vi "Teste Substrato Flexível 0.1_2022.vi"() -> ()   [LabVIEW 2016]
panel:
  out "F (Hz)":dbl format="%#_3g"
  out "Ciclos por segundo":dbl format="%#_3g"
  out "Tempo (s)":u32
  out "init":u32
  out "In LOOP":bool
  out "F2":bool
  out "F1":bool
  out "Close":bool
  out "Open":bool
  in  "Flush":bool
  in  "Loop Stop":i32=50 min=1
  in  "Loop Stop":bool
  in  "stop":bool
  in  "Loop Infinito":bool
  out "Vel Cte":i32
  in  "Vel Loop":i32(slide)=20 min=10 max=100 step=5 scale=10.0..100.0
  in  "Jog":i32=10
  in  "Jog_s":string="10"
  in  "Desl_s":string="50"
  out "Contador":dbl format="%.2f"
  in  "Power Off":bool
  in  "Down":bool
  in  "Up":bool
  out "read buffer":string
  out "Direcção":bool
  out "error":errorcluster
  in  "Arduino":refnum<visa-resource-name>="COM3"
  # "Controle Mecanismo Teste de Substrato Flexível"
  # "LOEM"
  # "Velocidade de Deslocamento"
  # "Contador de Ciclos"
  # "Parar em ciclo"
  # "CONTROLE MANUAL"
  # "Pg Up"
  # "Pg Down"
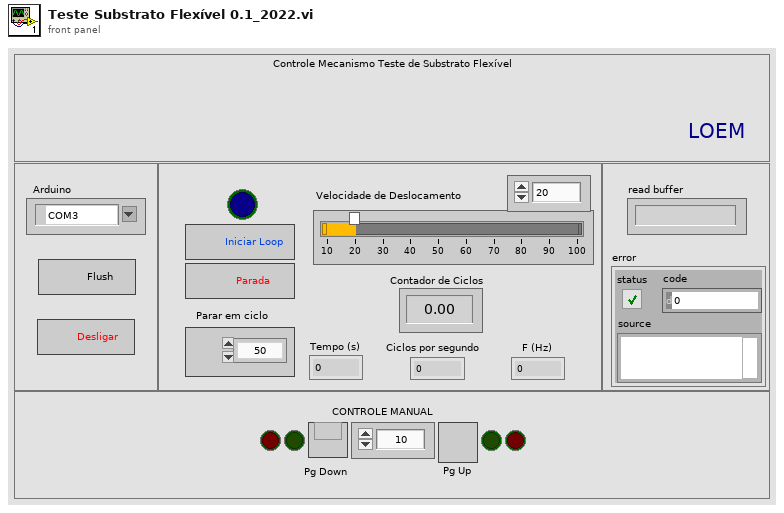
[diagram p1: front panel]
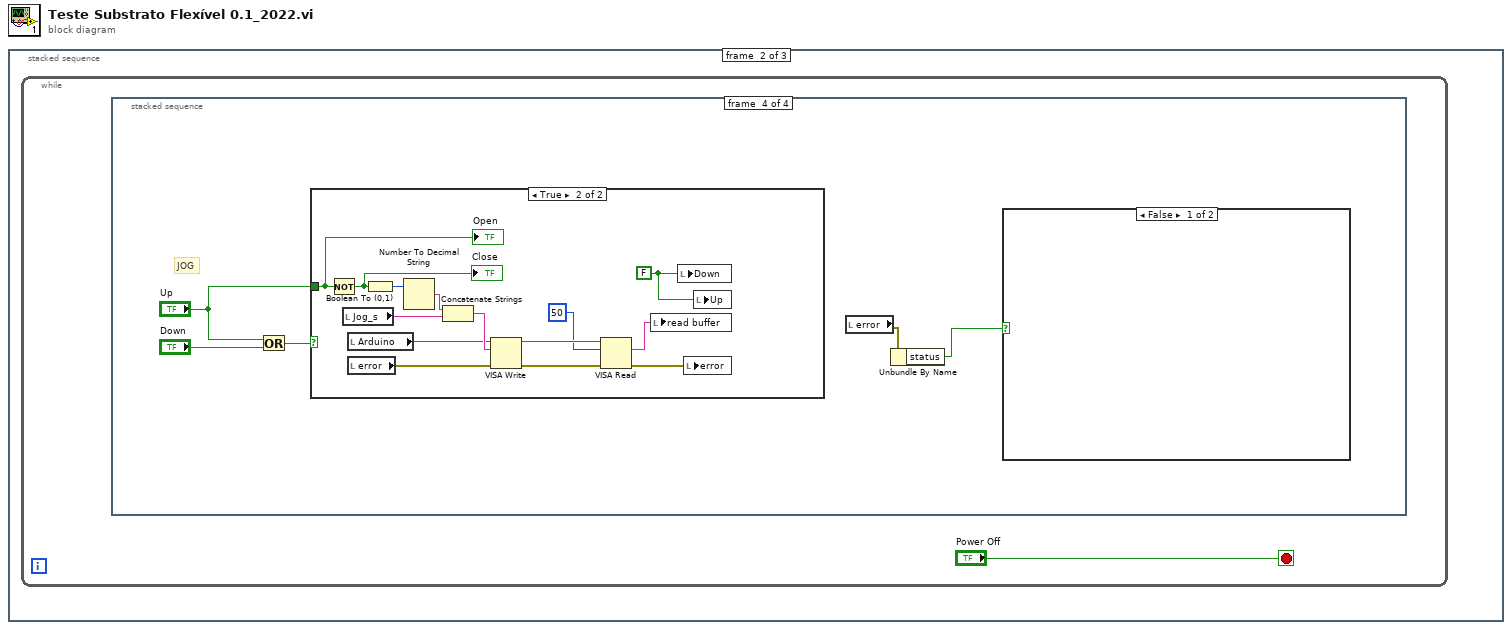
[diagram p0: block diagram]
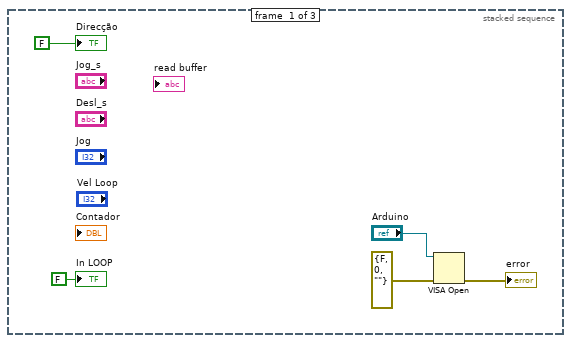
[diagram p2: hidden frame]
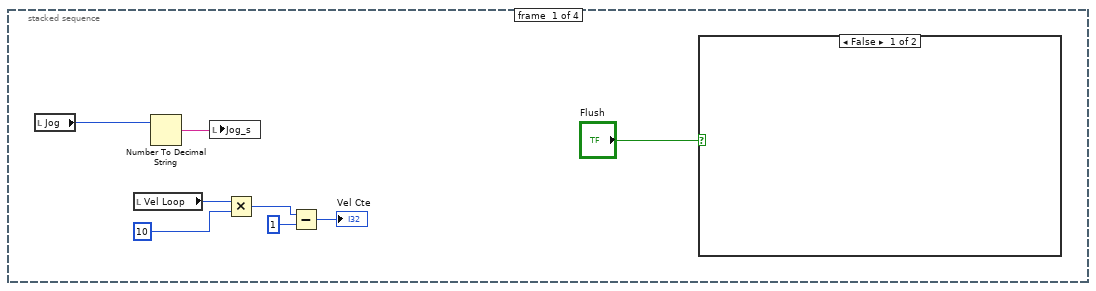
[diagram p3: hidden frame]
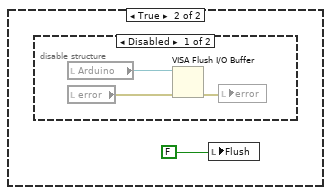
[diagram p4: hidden frame]
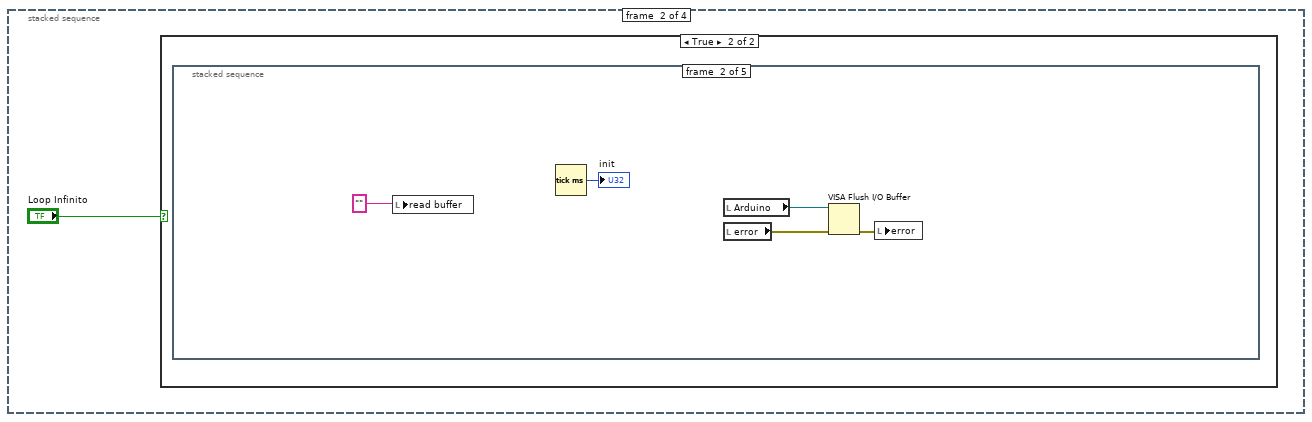
[diagram p6: hidden frame]
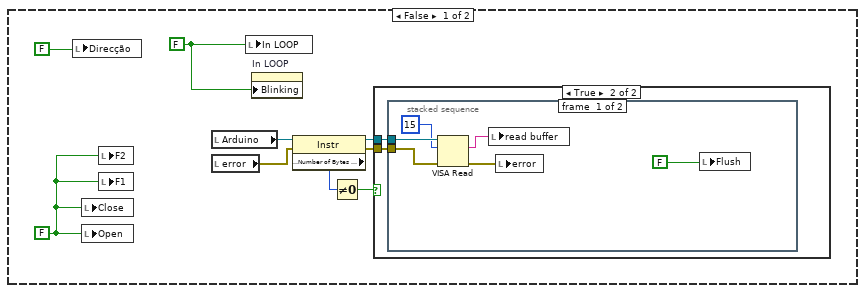
[diagram p7: hidden frame]
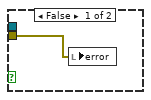
[diagram p8: hidden frame]
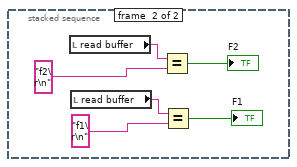
[diagram p9: hidden frame]
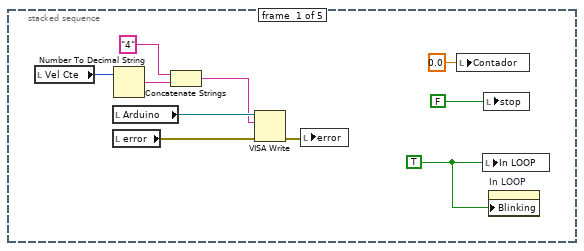
[diagram p10: hidden frame]
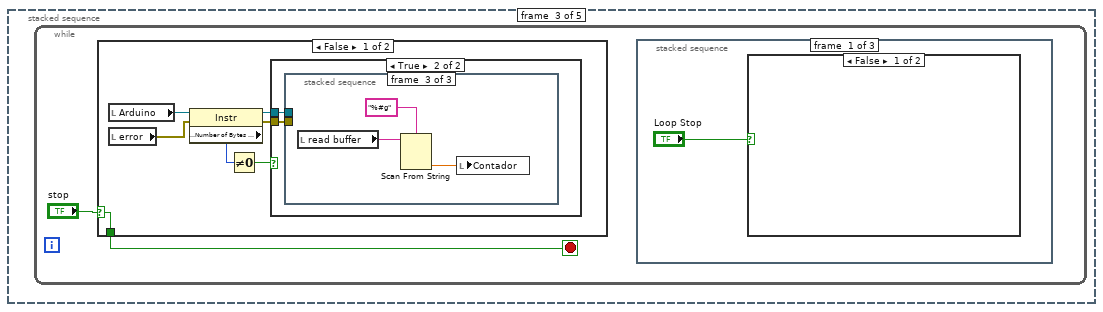
[diagram p11: hidden frame]
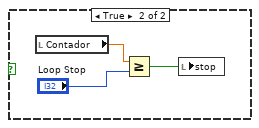
[diagram p12: hidden frame]
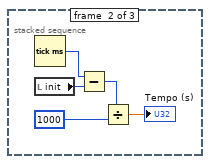
[diagram p13: hidden frame]
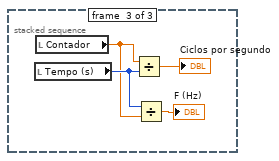
[diagram p14: hidden frame]
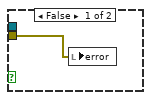
[diagram p15: hidden frame]
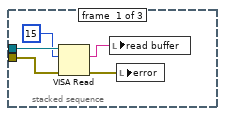
[diagram p16: hidden frame]
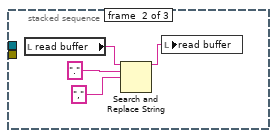
[diagram p17: hidden frame]
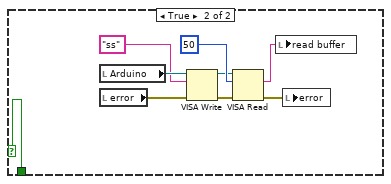
[diagram p18: hidden frame]
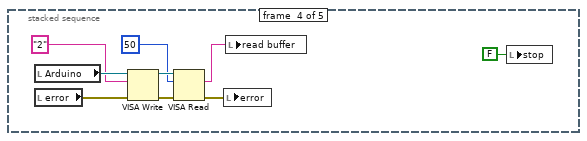
[diagram p19: hidden frame]
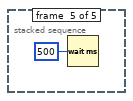
[diagram p20: hidden frame]
diagram:
  n1 = stacked-sequence {
    frame #0 {
      n2 = VISA Open(error in (no error)=errorcluster {"status"=FALSE, "code"=0, "source"=""}, VISA resource name="Arduino") -> (error out=→"error":errorcluster)  [unwired: 3 in, 1 out]
      "Direcção" <- FALSE ("Direcção")
      "In LOOP" <- FALSE ("In LOOP")
    }
    frame #1 {
      n3 = while {
        stop <- "Power Off" stop-if-true
        n4 = stacked-sequence {
          frame #0 {
            n5 = local read "Jog"() -> (w14:i32)
            n6 = local read "Vel Loop"() -> (w11:i32)
            n7 = Number To Decimal String(number=w14) -> (decimal integer string=w13:string)  [unwired: 1 in]
            n8 = local write "Jog_s"(w13) -> ()
            n9 = Multiply(x=w11, y=10) -> (x*y=w12:i32)
            n10 = Subtract(x=w12, y=1) -> (x-y=→"Vel Cte":i32)
            n11 = case shown="False" "Flush" {
              frame False {
              }
              frame True {
                n12 = disable-structure shown="Disabled" {
                  frame Disabled {
                    n13 = local read "Arduino"() -> (w16:refnum<visa-resource-name>)
                    n14 = local read "error"() -> (w17:errorcluster)
                    n15 = VISA Flush I/O Buffer(VISA resource name=w16, error in (no error)=w17) -> (error out=w18:errorcluster)  [unwired: 1 in, 1 out]
                    n16 = local write "error"(w18) -> ()
                  }
                  frame Enabled {
                  }
                }
                n17 = local write "Flush"(FALSE ("Direcção")) -> ()
              }
            }
          }
          frame #1 {
            n18 = case shown="True" "Loop Infinito" {
              frame False {
                w20 = FALSE ("In LOOP")
                w21 = FALSE ("Open")
                n19 = local write "Direcção"(FALSE ("Direcção")) -> ()
                n20 = local write "Close"(w21) -> ()
                n21 = local write "Open"(w21) -> ()
                n22 = local write "F2"(w21) -> ()
                n23 = local write "F1"(w21) -> ()
                n24 = local read "Arduino"() -> (w22:refnum<visa-resource-name>)
                n25 = local read "error"() -> (w24:errorcluster)
                n26 = local write "In LOOP"(w20) -> ()
                n27 = property on="In LOOP" class="Bool (strict)"("Blinking"=w20) -> ()  [unwired: 2 in, 2 out]
                n28 = property class="Instr"(reference=w22, error in=w24) -> (reference out=w23:refnum<visa-resource-name>, error out=w25:errorcluster, "Serial Settings:Number of Bytes at Serial Port"=w27:u32)
                n29 = Not Equal To 0?(x=w27) -> (x != 0?=w26:bool)
                n30 = case shown="True" w26 {
                  tunnel: w23 -> [_ w31]
                  tunnel: w25 -> [w29 w30]
                  frame False {
                    n31 = local write "error"(w29) -> ()
                  }
                  frame True {
                    n32 = stacked-sequence {
                      tunnel: w31 -> [w36 _]
                      tunnel: w30 -> [w34 _]
                      frame #0 {
                        n33 = VISA Read(VISA resource name=w36, byte count=u32 15, error in (no error)=w34) -> (read buffer=w33:string, error out=w37:errorcluster)  [unwired: 2 out]
                        n34 = local write "read buffer"(w33) -> ()
                        n35 = local write "error"(w37) -> ()
                        n36 = local write "Flush"(FALSE ("Direcção")) -> ()
                      }
                      frame #1 {
                        n37 = local read "read buffer"() -> (w40:string)
                        n38 = local read "read buffer"() -> (w42:string)
                        n39 = Equal?(x=w40, y="f2\r\n" ("read buffer")) -> (x = y?=→"F2":bool)
                        n40 = Equal?(x=w42, y="f1\r\n" ("read buffer")) -> (x = y?=→"F1":bool)
                      }
                    }
                  }
                }
              }
              frame True {
                n41 = stacked-sequence {
                  frame #0 {
                    w44 = TRUE ("In LOOP")
                    n42 = local read "Vel Cte"() -> (w45:i32)
                    n43 = local read "Arduino"() -> (w51:refnum<visa-resource-name>)
                    n44 = local read "error"() -> (w52:errorcluster)
                    n45 = Number To Decimal String(number=w45) -> (decimal integer string=w48:string)  [unwired: 1 in]
                    n46 = Concatenate Strings("4" ("write buffer"), w48) -> (w50:string)
                    n47 = VISA Write(VISA resource name=w51, write buffer=w50, error in (no error)=w52) -> (error out=w53:errorcluster)  [unwired: 2 out]
                    n48 = local write "error"(w53) -> ()
                    n49 = local write "Contador"(0.0 ("Contador")) -> ()
                    n50 = local write "In LOOP"(w44) -> ()
                    n51 = local write "stop"(FALSE ("stop")) -> ()
                    n52 = property on="In LOOP" class="Bool (strict)"("Blinking"=w44) -> ()  [unwired: 2 in, 2 out]
                  }
                  frame #1 {
                    n53 = local write "read buffer"("" ("read buffer")) -> ()
                    n54 = Tick Count (ms)() -> (millisecond timer value=→"init":u32)
                    n55 = local read "Arduino"() -> (w56:refnum<visa-resource-name>)
                    n56 = local read "error"() -> (w57:errorcluster)
                    n57 = VISA Flush I/O Buffer(VISA resource name=w56, error in (no error)=w57) -> (error out=w58:errorcluster)  [unwired: 1 in, 1 out]
                    n58 = local write "error"(w58) -> ()
                  }
                  frame #2 {
                    n59 = while {
                      stop <- w59 stop-if-true
                      n60 = case shown="False" "stop" {
                        selector: "stop" -> [w80 w96]
                        tunnel: [w80 w96] -> w59
                        frame False {
                          n61 = local read "Arduino"() -> (w74:refnum<visa-resource-name>)
                          n62 = local read "error"() -> (w76:errorcluster)
                          n63 = property class="Instr"(reference=w74, error in=w76) -> (reference out=w75:refnum<visa-resource-name>, error out=w77:errorcluster, "Serial Settings:Number of Bytes at Serial Port"=w79:u32)
                          n64 = Not Equal To 0?(x=w79) -> (x != 0?=w78:bool)
                          n65 = case shown="True" w78 {
                            tunnel: w75 -> [_ w83]
                            tunnel: w77 -> [w81 w82]
                            frame False {
                              n66 = local write "error"(w81) -> ()
                            }
                            frame True {
                              n67 = stacked-sequence {
                                tunnel: w83 -> [w87 _ _]
                                tunnel: w82 -> [w85 _ _]
                                frame #0 {
                                n68 = VISA Read(VISA resource name=w87, byte count=u32 15, error in (no error)=w85) -> (read buffer=w84:string, error out=w88:errorcluster)  [unwired: 2 out]
                                n69 = local write "read buffer"(w84) -> ()
                                n70 = local write "error"(w88) -> ()
                                }
                                frame #1 {
                                n71 = local read "read buffer"() -> (w92:string)
                                n72 = Search and Replace String(input string=w92, search string=".", replace string="," ("replace string (\"\")")) -> (result string=w91:string)  [unwired: 5 in, 3 out]
                                n73 = local write "read buffer"(w91) -> ()
                                }
                                frame #2 {
                                n74 = local read "read buffer"() -> (w95:string)
                                n75 = Scan From String(format string="%#g", input string=w95) -> (output 1=w93:dbl)  [unwired: 3 in, 3 out]
                                n76 = local write "Contador"(w93) -> ()
                                }
                              }
                            }
                          }
                        }
                        frame True {
                          n77 = local read "Arduino"() -> (w104:refnum<visa-resource-name>)
                          n78 = local read "error"() -> (w103:errorcluster)
                          n79 = VISA Write(VISA resource name=w104, write buffer="ss", error in (no error)=w103) -> (VISA resource name out=w99:refnum<visa-resource-name>, error out=w101:errorcluster)  [unwired: 1 out]
                          n80 = VISA Read(VISA resource name=w99, byte count=u32 50, error in (no error)=w101) -> (read buffer=w97:string, error out=w102:errorcluster)  [unwired: 2 out]
                          n81 = local write "read buffer"(w97) -> ()
                          n82 = local write "error"(w102) -> ()
                        }
                      }
                      n83 = stacked-sequence {
                        frame #0 {
                          n84 = case shown="False" "Loop Stop" {
                            frame False {
                            }
                            frame True {
                              n85 = local read "Contador"() -> (w64:dbl)
                              n86 = Greater Or Equal?(x=w64, y="Loop Stop") -> (x >= y?=w62:bool)
                              n87 = local write "stop"(w62) -> ()
                            }
                          }
                        }
                        frame #1 {
                          n88 = Tick Count (ms)() -> (millisecond timer value=w68:u32)
                          n89 = local read "init"() -> (w69:u32)
                          n90 = Subtract(x=w68, y=w69) -> (x-y=w67:u32)
                          n91 = Divide(x=w67, y=u32 1000) -> (x/y=→"Tempo (s)":dbl)
                        }
                        frame #2 {
                          n92 = local read "Tempo (s)"() -> (w72:u32)
                          n93 = local read "Contador"() -> (w71:dbl)
                          n94 = Divide(x=w71, y=w72) -> (x/y=→"Ciclos por segundo":dbl)
                          n95 = Divide(x=w72, y=w71) -> (x/y=→"F (Hz)":dbl)
                        }
                      }
                    }
                  }
                  frame #3 {
                    n96 = local read "Arduino"() -> (w109:refnum<visa-resource-name>)
                    n97 = local read "error"() -> (w110:errorcluster)
                    n98 = VISA Write(VISA resource name=w109, write buffer="2", error in (no error)=w110) -> (VISA resource name out=w113:refnum<visa-resource-name>, error out=w112:errorcluster)  [unwired: 1 out]
                    n99 = VISA Read(VISA resource name=w113, byte count=u32 50, error in (no error)=w112) -> (read buffer=w108:string, error out=w111:errorcluster)  [unwired: 2 out]
                    n100 = local write "error"(w111) -> ()
                    n101 = local write "read buffer"(w108) -> ()
                    n102 = local write "stop"(FALSE ("stop")) -> ()
                  }
                  frame #4 {
                    n103 = Wait (ms)(milliseconds to wait=u32 500) -> ()  [unwired: 1 out]
                  }
                }
              }
            }
          }
          frame #2 {
            n104 = local read "stop"() -> (w115:bool)
            n105 = case shown="True" w115 {
              frame False {
              }
              frame True {
                n106 = local read "Arduino"() -> (w118:refnum<visa-resource-name>)
                n107 = local read "error"() -> (w119:errorcluster)
                n108 = VISA Write(VISA resource name=w118, write buffer="ss", error in (no error)=w119) -> (VISA resource name out=w123:refnum<visa-resource-name>, error out=w121:errorcluster)  [unwired: 1 out]
                n109 = VISA Read(VISA resource name=w123, byte count=u32 50, error in (no error)=w121) -> (read buffer=w125:string, error out=w120:errorcluster)  [unwired: 2 out]
                n110 = local write "read buffer"(w125) -> ()
                n111 = local write "error"(w120) -> ()
                n112 = local write "stop"(FALSE ("stop")) -> ()
              }
            }
            n113 = Wait (ms)(milliseconds to wait=u32 150) -> ()  [unwired: 1 out]
          }
          frame #3 {
            # "JOG"
            n114 = Or(x="Up", y="Down") -> (x .or. y?=w129:bool)
            n115 = case shown="True" w129 {
              tunnel: "Up" -> [_ w139]
              frame False {
              }
              frame True {
                w141 = FALSE ("Previous")
                n116 = Not(x=w139) -> (.not. x?=w138:bool)
                "Close" <- w138
                n117 = local read "Jog_s"() -> (w140:string)
                n118 = local read "Arduino"() -> (w144:refnum<visa-resource-name>)
                n119 = local read "error"() -> (w145:errorcluster)
                n120 = Boolean To (0,1)(Boolean=w138) -> (0, 1=w148:i16)
                n121 = Number To Decimal String(number=w148) -> (decimal integer string=w149:string)  [unwired: 1 in]
                n122 = Concatenate Strings(w149, w140) -> (w147:string)
                n123 = VISA Write(VISA resource name=w144, write buffer=w147, error in (no error)=w145) -> (VISA resource name out=w151:refnum<visa-resource-name>, error out=w150:errorcluster)  [unwired: 1 out]
                n124 = VISA Read(VISA resource name=w151, byte count=u32 50, error in (no error)=w150) -> (read buffer=w143:string, error out=w146:errorcluster)  [unwired: 2 out]
                n125 = local write "read buffer"(w143) -> ()
                n126 = local write "Down"(w141) -> ()
                n127 = local write "error"(w146) -> ()
                n128 = local write "Up"(w141) -> ()
                "Open" <- w139
              }
            }
            n129 = local read "error"() -> (w127:errorcluster)
            n130 = Unbundle By Name(w127) -> ("status"=w126:bool)
            n131 = case shown="False" w126 {
              frame False {
              }
              frame True {
                n132 = stacked-sequence {
                  frame #0 {
                    n133 = local read "Arduino"() -> (w131:refnum<visa-resource-name>)
                    n134 = local read "error"() -> (w132:errorcluster)
                    n135 = VISA Close(VISA resource name=w131, error in (no error)=w132) -> (error out=w133:errorcluster)
                    n136 = local write "error"(w133) -> ()
                  }
                  frame #1 {
                    n137 = Wait (ms)(milliseconds to wait=u32 200) -> ()  [unwired: 1 out]
                  }
                  frame #2 {
                    n138 = local read "Arduino"() -> (w136:refnum<visa-resource-name>)
                    n139 = VISA Open(error in (no error)=errorcluster {"status"=FALSE, "code"=0, "source"=""}, VISA resource name=w136) -> (error out=w137:errorcluster)  [unwired: 3 in, 1 out]
                    n140 = local write "error"(w137) -> ()
                  }
                }
              }
            }
          }
        }
      }
    }
    frame #2 {
      n141 = local read "Arduino"() -> (w154:refnum<visa-resource-name>)
      n142 = local read "error"() -> (w153:errorcluster)
      n143 = VISA Close(VISA resource name=w154, error in (no error)=w153) -> (error out=w152:errorcluster)
      n144 = local write "error"(w152) -> ()
    }
  }
